vi "BasicLoginPanel.vi"() -> ()   [LabVIEW 2019]
panel:
  in  "Submit":bool
  in  "Password":string
  in  "Username":string
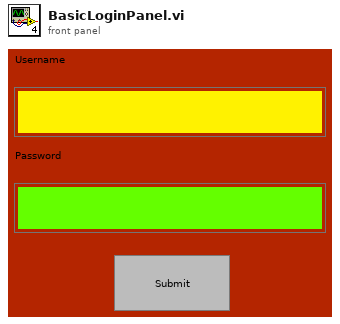
[diagram p1: front panel]
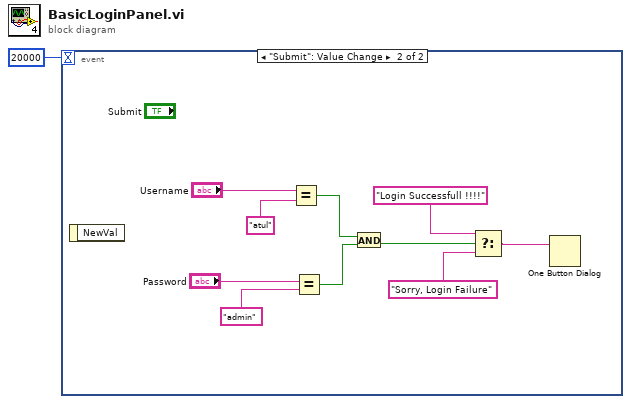
[diagram p0: block diagram]
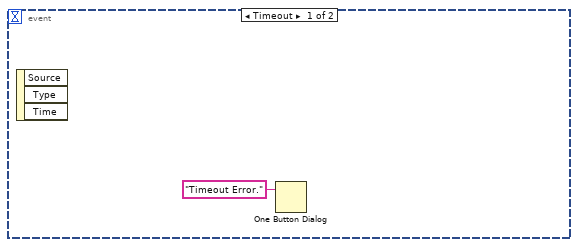
[diagram p2: hidden frame]
diagram:
  n1 = event shown="[1] \"Submit\": Value Change" {
    selector: _ -> [_ _]
    dyn-events: _ -> [_ _]
    timeout: 20000 -> [_ _]
    event Timeout {
      n2 = event-data() -> ()  [unwired: 1 in, 3 out]
      n3 = One Button Dialog(message="Timeout Error.") -> ()  [unwired: 1 in, 1 out]
    }
    event "Submit": Value Change {
      n4 = event-data() -> ()  [unwired: 1 in, 1 out]
      n5 = Equal?(x="Username", y="atul") -> (x = y?=w8:bool)
      n6 = Equal?(x="Password", y="admin") -> (x = y?=w7:bool)
      n7 = And(x=w8, y=w7) -> (x .and. y?=w6:bool)
      n8 = Select(t="Login Successfull !!!!", s=w6, f="Sorry, Login Failure") -> (s? t:f=w3:string)
      n9 = One Button Dialog(message=w3) -> ()  [unwired: 1 in, 1 out]
    }
  }
